vi "File Popup For Save.vi"(8 "error in (no error)":errorcluster) -> (0 "error out":errorcluster, 2 "cancelled":bool, 3 "selected path":path)   [LabVIEW 2021]
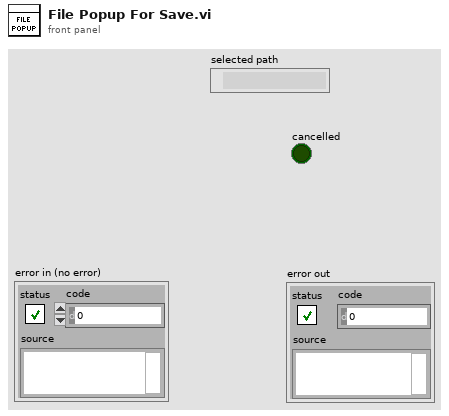
[diagram p1: front panel]
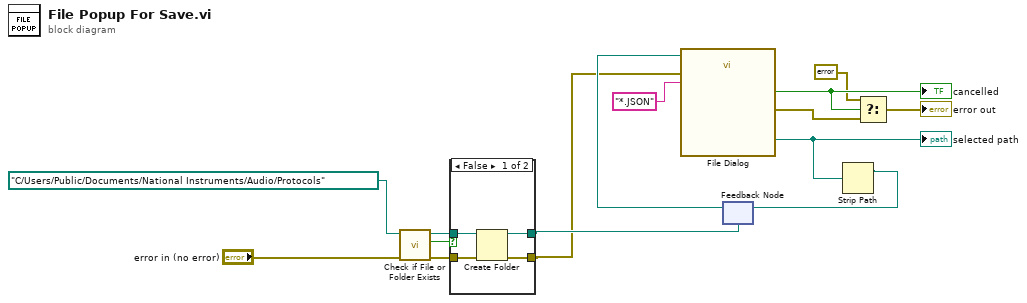
[diagram p0: block diagram]
diagram:
  n1 = call <vilib>:"Check if File or Folder Exists.vi"("error in (no error)"="error in (no error)", "path"=path "C:/Users/Public/Documents/National Instruments/Audio/Protocols") -> ("error out"=w14:errorcluster, "file or folder exists?"=w15:bool, "dup path"=w13:path)  [unwired: 7 in]
  n2 = case shown="False" w15 {
    tunnel: w14 -> [w19 w20]
    tunnel: w13 -> [w18 w21]
    tunnel: [w17 w21] -> w8
    tunnel: [w16 w20] -> w6
    frame False {
      n3 = Create Folder(path (use dialog)=w18, error in=w19) -> (created path=w17:path, error out=w16:errorcluster)  [unwired: 1 in, 1 out]
    }
    frame True {
    }
  }
  n4 = feedback #1(w8) -> (w7:path)
  n5 = call "File Dialog"("start path"=w7, "error in"=w6, "pattern (all files)"="*.JSON") -> ("selected path"=w10:path, "cancelled"=w5:bool, "error out"=w4:errorcluster)  [unwired: 9 in, 1 out]
  "cancelled" <- w5
  "selected path" <- w10
  n6 = Strip Path(path=w10) -> (stripped path=w9:path)  [unwired: 1 out]
  n7 = feedback-in #1(w9) -> ()
  n8 = Select(t=errorcluster {"status"=FALSE, "code"=0, "source"=""}, s=w5, f=w4) -> (s? t:f=→"error out":errorcluster)
